vi "Offset Inline Buffers.vi"(8 "error in (no error)":errorcluster, 10 "Engine Pointer":refnum<class "Memory.Pointer.lvclass">, 11 "Transfer Group in":refnum<class "Transfer Group.lvclass">) -> (0 "error out":errorcluster, 3 "Transfer Group out":refnum<class "Transfer Group.lvclass">)   [LabVIEW 2017, in "Data Sharing Framework Core.lvlib" / "Data Sharing Framework Engine.lvlib" / "Transfer Group.lvclass"]
uses:
  Transfer Group.lvclass
  <vilib>/National Instruments/Memory Manager/Classes/Pointer/Memory.Pointer.lvclass
  Transfer Group.lvclass/Transfer Group.ctl
  Transfer/Transfer.lvclass
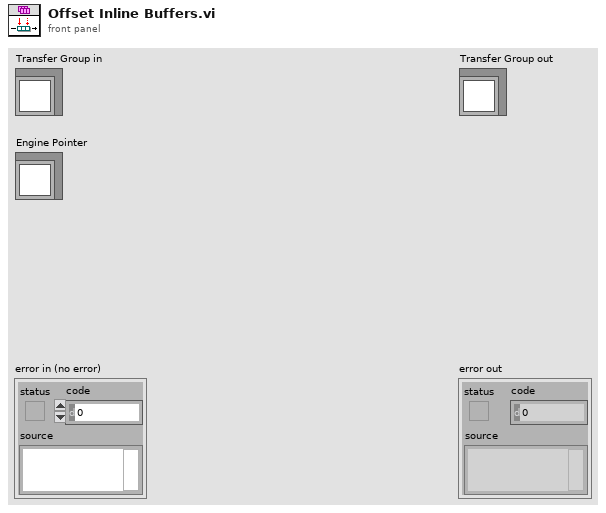
[diagram p1: front panel]
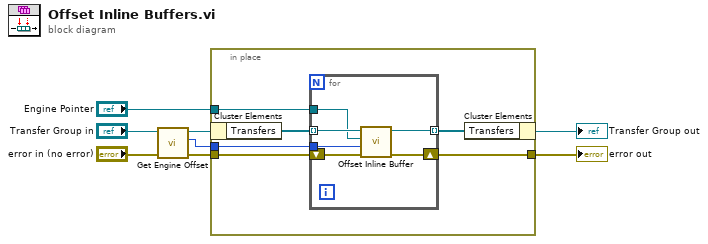
[diagram p0: block diagram]
diagram:
  n1 = call "Get Engine Offset.vi"("Transfer Group in"="Transfer Group in") -> ("engine offset"=w2:u64, "Transfer Group out"=w3:refnum<class "Transfer Group.lvclass">)  [unwired: 9 in]
  n2 = in-place {
    in-place-border: [w11] -> w7
    in-place-border: "error in (no error)" -> [w10]
    in-place-border: "Engine Pointer" -> [w9]
    in-place-border: w2 -> [w8]
    n3 = in-place-cluster #1(w3) -> ("Transfers"=w13:refnum<class "Transfer.lvclass">[])
    n4 = for {
      tunnel: w13 -> [w19] mode=indexing
      tunnel: [w18] -> w12 mode=indexing
      shift-right: [w17] -> w11
      shift-left: w10 -> [w16]
      tunnel: w9 -> [w14]
      tunnel: w8 -> [w15]
      n5 = call "Offset Inline Buffer.vi"("error in (no error)"=w16, "group engine offset"=w15, "Engine Pointer"=w14, "Transfer in"=w19) -> ("error out"=w17:errorcluster, "Transfer out"=w18:refnum<class "Transfer.lvclass">)  [unwired: 6 in]
    }
    n6 = in-place-cluster #1("Transfers"=w12) -> (→"Transfer Group out":refnum<class "Transfer Group.lvclass">)
  }
  "error out" <- w7
